vi "_save_csv_InPhaseStep.vi"(6 "Method":u16(ring)=1 items=["dBm"=1, "mW"=2], 7 "delimiter (\\t)":string="SingleCh_", 11 "dataInput":string[][](array[string])) -> (3 "FileName":string)   [LabVIEW 2023]
uses:
  <vilib>/Utility/file.llb/Write Delimited Spreadsheet (string).vi
panel:
  out "appended path":path
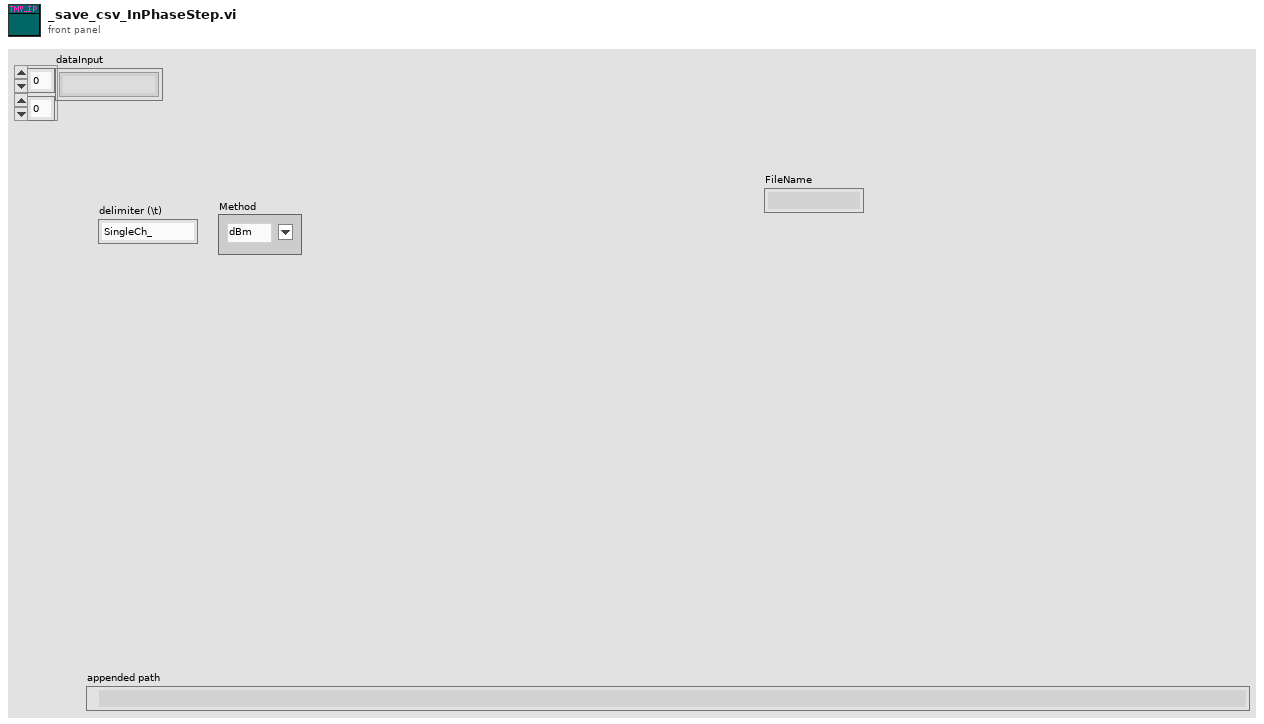
[diagram p1: front panel]
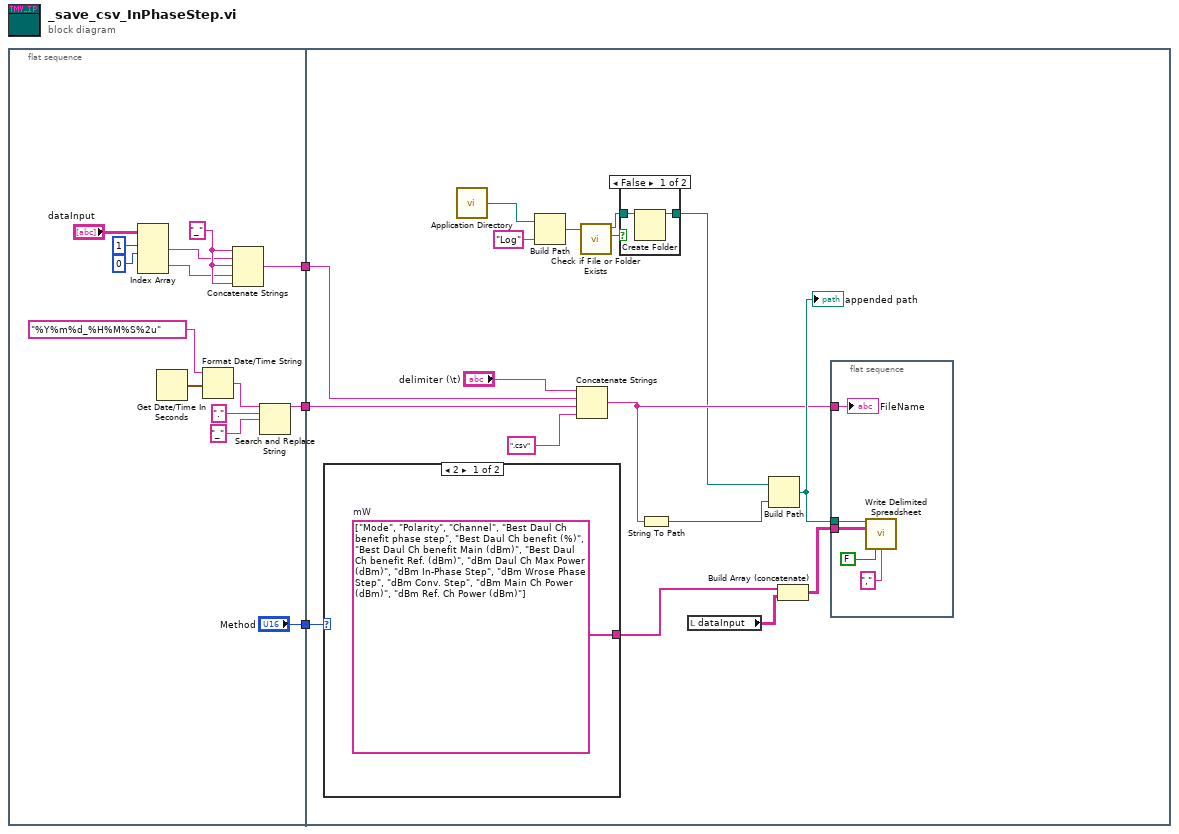
[diagram p0: block diagram]
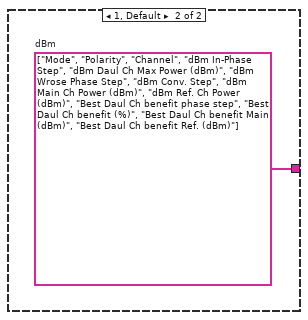
[diagram p3: hidden frame]
diagram:
  n1 = flat-sequence {
    tunnel: [w12] -> w3
    tunnel: ["Method"] -> w2
    tunnel: [w4] -> w1
    tunnel: w3 -> [w26]
    tunnel: w2 -> [w25]
    tunnel: w1 -> [w23]
    frame #0 {
      w7 = "_"
      n2 = Index Array(array="dataInput", index (row) #1=1 ("index (row)"), index (col) #1=0 ("disabled index (col)")) -> (element #1=w6:string, element #2=w5:string)  [unwired: 2 in]
      n3 = Get Date/Time In Seconds() -> (seconds since 1Jan1904=w17:timestamp)
      n4 = Format Date/Time String(time format string (%c)="%Y%m%d_%H%M%S%2u", seconds (now)=w17) -> (date/time string=w15:string)  [unwired: 1 in]
      n5 = Concatenate Strings(w7, w6, w7, w5, w7) -> (w4:string)
      n6 = Search and Replace String(input string=w15, search string=".", replace string="_") -> (result string=w12:string)  [unwired: 5 in, 3 out]
    }
    frame #1 {
      n7 = case shown="2" w25 {
        tunnel: [w38 w39] -> w30
        frame 2 {
          w38 = string[] ["Mode", "Polarity", "Channel", "Best Daul Ch benefit phase step", "Best Daul Ch benefit (%)", "Best Daul Ch benefit Main (dBm)", "Best Daul Ch benefit Ref. (dBm)", "dBm Daul Ch Max Power (dBm)", "dBm In-Phase Step", "dBm Wrose Phase Step", "dBm Conv. Step", "dBm Main Ch Power (dBm)", "dBm Ref. Ch Power (dBm)"]  # mW
        }
        frame 1, Default {
          w39 = string[] ["Mode", "Polarity", "Channel", "dBm In-Phase Step", "dBm Daul Ch Max Power (dBm)", "dBm Wrose Phase Step", "dBm Conv. Step", "dBm Main Ch Power (dBm)", "dBm Ref. Ch Power (dBm)", "Best Daul Ch benefit phase step", "Best Daul Ch benefit (%)", "Best Daul Ch benefit Main (dBm)", "Best Daul Ch benefit Ref. (dBm)"]  # dBm
        }
      }
      n8 = call <vilib>:"Application Directory.vi"() -> ("Application Directory"=w28:path)
      n9 = Build Path(base path=w28, name or relative path="Log") -> (appended path=w19:path)
      n10 = Concatenate Strings("delimiter (\\t)", w23, w26, ".csv" ("delimiter (\\t)")) -> (w31:string)
      n11 = call <vilib>:"Check if File or Folder Exists.vi"("path"=w19) -> ("file or folder exists?"=w21:bool, "dup path"=w20:path)  [unwired: 8 in, 1 out]
      n12 = case shown="False" w21 {
        tunnel: w20 -> [w36 w37]
        tunnel: [w35 w37] -> w18
        frame False {
          n13 = Create Folder(path (use dialog)=w36) -> (created path=w35:path)  [unwired: 2 in, 2 out]
        }
        frame True {
        }
      }
      n14 = String To Path(string=w31) -> (path=w33:path)
      n15 = local read "dataInput"() -> (w22:string[][])
      n16 = Build Path(base path=w18, name or relative path=w33) -> (appended path=w32:path)
      "appended path" <- w32
      n17 = Build Array (concatenate)(w30, w22) -> (w29:string[][])
      n18 = flat-sequence {
        tunnel: w32 -> [w43]
        tunnel: w31 -> [w41]
        tunnel: w29 -> [w40]
        frame #0 {
          n19 = call-poly <vilib>:"Write Delimited Spreadsheet.vi"("file path (dialog if empty)"=w43, "2D data"=w40, "transpose? (no:F)"=FALSE, "delimiter (\\t)"="," ("delimiter (\\t)")) -> ()  [unwired: 10 in, 2 out]
          "FileName" <- w41
        }
      }
    }
  }
